vi "Get Volts.vi"(8 "error in (no error)":errorcluster, 11 "Instrumento feo in":refnum<class "Instrumento feo.lvclass">) -> (0 "error out":errorcluster, 2 "Volts":dbl, 3 "Instrumento feo out":refnum<class "Instrumento feo.lvclass">)   [LabVIEW 2020, in "Instrumento feo.lvclass"]
uses:
  Instrumento feo.lvclass
  Instrumento feo.lvclass/Instrumento feo.ctl
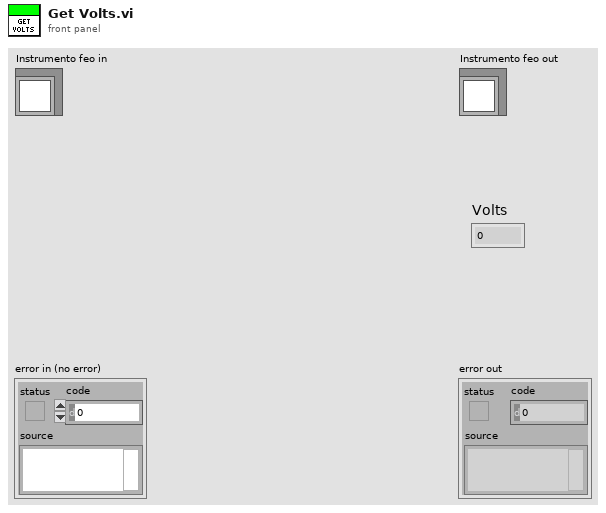
[diagram p1: front panel]
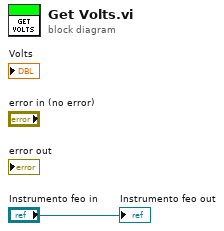
[diagram p0: block diagram]
diagram:
  "Instrumento feo out" <- "Instrumento feo in"
